vi "Begin.vi"(8 "error in":errorcluster) -> (0 "error out":errorcluster)   [LabVIEW 2017]
doc: "Called before other user functions, this VI is expected to open initial I/O refnums, load in file data, and do all program initialization. Notice that the <B>error out</B> terminal is simply used for data flow. Wiring it to other structures or subVIs ensures that this VI runs first."
uses:
  <vilib>/Rock Robotics/WPI/DriverStation/WPI_DriverStationRobotMode2.ctl
  <vilib>/Rock Robotics/WPI/Joystick/WPI_JoystickDeviceEnum.ctl
  <vilib>/Rock Robotics/WPI/Solenoid/WPI_SolenoidChannel.ctl
  <vilib>/Rock Robotics/SystemInterfaces/spilib/spi_bus.ctl
  C:/Users/Public/Documents/Cross The Road Electronics/Phoenix-LabVIEW/Motor Controller/Controls/CTRE_Phoenix_MotorControl_ControlMode.ctl
  <vilib>/Rock Robotics/WPI/ThirdParty/Phoenix-LabVIEW/Motor Controller/Controls/CTRE_Phoenix_MotorControl_NeutralMode.ctl
  <vilib>/Rock Robotics/WPI/ThirdParty/Phoenix-LabVIEW/Motor Controller/Controls/CTRE_Phoenix_MotorControl_FeedbackDevice.ctl
  <vilib>/Rock Robotics/SystemInterfaces/DIO/FPGA_DIOChannel.ctl
  <vilib>/Rock Robotics/SystemInterfaces/AI/FPGA_AIChannel.ctl
  Robot Global Data.vi
  <vilib>/Rock Robotics/WPI/Solenoid/WPI_SolenoidOpenDouble.vi
  <vilib>/Rock Robotics/WPI/Solenoid/WPI_SolenoidOpenSingle.vi
  <vilib>/Rock Robotics/WPI/Switch/WPI_SwitchOpenLimit.vi
  <vilib>/Rock Robotics/WPI/Gyro/WPI_GyroXRS450_SPI_Open.vi
  <vilib>/Rock Robotics/Network Tables/NT Write Numeric Array.vi
  <vilib>/Rock Robotics/Network Tables/NT Write String Array.vi
panel:
  in  "Right_P":dbl
  in  "Right_I":dbl
  in  "Right_D":dbl
  in  "Right_F":dbl
  in  "Left_F":dbl
  in  "Left_D":dbl
  in  "Left_I":dbl
  in  "Left_P":dbl
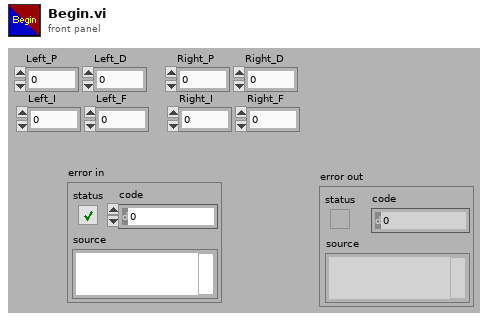
[diagram p1: front panel]
types:
  T1 = typedef "FPGA_AIChannel.ctl" = enum8{"AI 0", "AI 1", "AI 2", "AI 3", "AI MXP 0", "AI MXP 1", "AI MXP 2", "AI MXP 3", "Invalid"}
  T2 = typedef "FPGA_DIOChannel.ctl" = enum8{"DIO 0", "DIO 1", "DIO 2", "DIO 3", "DIO 4", "DIO 5", "DIO 6", "DIO 7", "DIO 8", "DIO 9", "DIO MXP 0", "DIO MXP 1", "DIO MXP 2", "DIO MXP 3", "DIO MXP 4", "DIO MXP 5", "DIO MXP 6", "DIO MXP 7", "DIO MXP 8", "DIO MXP 9", "DIO MXP 10", "DIO MXP 11", "DIO MXP 12", "DIO MXP 13", "DIO MXP 14", "DIO MXP 15", "SPI Port CS1", "SPI Port CS2", "SPI Port CS3", "SPI Port MISO", "SPI Port MOSI", "Invalid"}
  T3 = typedef "CTRE_Phoenix_MotorControl_FeedbackDevice.ctl" = i8
  T4 = typedef "CTRE_Phoenix_MotorControl_NeutralMode.ctl" = enum8{"EEPROMSetting", "Override to Coast", "Override to Brake"}
  T5 = typedef "CTRE_Phoenix_MotorControl_ControlMode.ctl" = u16
  T6 = typedef "spi_bus.ctl" = enum16{"SPI On-Board, CS0", "SPI On-Board, CS1", "SPI On-Board, CS2", "SPI On-Board, CS3", "SPI MXP", "Invalid"}
  T7 = typedef "WPI_SolenoidChannel.ctl" = enum8{"Solenoid 0", "Solenoid 1", "Solenoid 2", "Solenoid 3", "Solenoid 4", "Solenoid 5", "Solenoid 6", "Solenoid 7", "Invalid"}
  T8 = typedef "WPI_JoystickDeviceEnum.ctl" = enum16{"USB 0", "USB 1", "USB 2", "USB 3", "USB 4", "USB 5"}
  T9 = typedef "WPI_DriverStationRobotMode2.ctl" = enum16{"Autonomous Disabled", "Autonomous Enabled", "Teleop Disabled", "Teleop Enabled", "Disconnected", "Finish", "Test Disabled", "Test Enabled", "Emergency Stopped"}
  T10 = typedef "WPI_MotorControlDeviceRef.ctl" = cluster{"DeviceStatus":errorcluster, "Type":T11, "PWM":cluster{"PWM Channel":T12, "DeadBand":T13}, "CAN":cluster{"Device Number":u8, "SetOutput VI Ref":variant, "GetOutput VI Ref":variant, "Enable VI Ref":variant, "Disable VI Ref":variant, "Data":variant}, "Invert":bool, "DIO PWM":cluster{"PWM \"Enable\" Channel":T12, "DIOChannel":T2, "PWM Rate":dbl}}
  T11 = typedef "WPI_MotorControlType.ctl" = enum16{"PWM", "CAN", "DIO PWM"}
  T12 = typedef "FPGA_DIOPWMChannel.ctl" = enum8{"PWM 0", "PWM 1", "PWM 2", "PWM 3", "PWM 4", "PWM 5", "PWM 6", "PWM 7", "PWM 8", "PWM 9", "PWM MXP 0", "PWM MXP 1", "PWM MXP 2", "PWM MXP 3", "PWM MXP 4", "PWM MXP 5", "PWM MXP 6", "PWM MXP 7", "PWM MXP 8", "PWM MXP 9", "Invalid"}
  T13 = typedef "WPI_PWMDeadband.ctl" = cluster{"Name":string, "maxPositivePwm":i32, "minPositivePwm":i32, "centerPwm":i32, "maxNegativePwm":i32, "minNegativePwm":i32, "angularRange":u16}
  T14 = typedef "WPI_SolenoidDevRef.ctl" = cluster{"DevStatus":errorcluster, "Pneumatics Control Module":u8, "Forward Solenoid Channel":T7, "Reverse Solenoid Channel":T7}
  T15 = typedef "WPI_JoystickDevRef.ctl" = cluster{"Device":T8}
  T16 = typedef "WPI_AnalogChannelDevRef.ctl" = cluster{"DevStatus":errorcluster, "Analog Channel":T1}
  T17 = typedef "WPI_SwitchDevRef.ctl" = cluster{"DevStatus":errorcluster, "DIO Channel":T2, "CntIndex":T18, "Normally Closed":bool}
  T18 = typedef "FPGA_CounterCtrSystemIndex.ctl" = enum8{"Ctr 0", "Ctr 1", "Ctr 2", "Ctr 3", "Ctr 4", "Ctr 5", "Ctr 6", "Ctr 7", "Invalid"}
  T19 = typedef "WPI_GyroDevRef.ctl" = cluster{"DevStatus":errorcluster, "Analog Channel":T1, "Gain (VoltsPerDegree/Second)":dbl, "Gyro Type":enum16{"Analog", "XRS450"}, "Handle":i32, "SPI Bus":T6, "Device Found":bool, "Sample Rate":dbl, "Calibrate On Open":bool, "Offset":dbl}
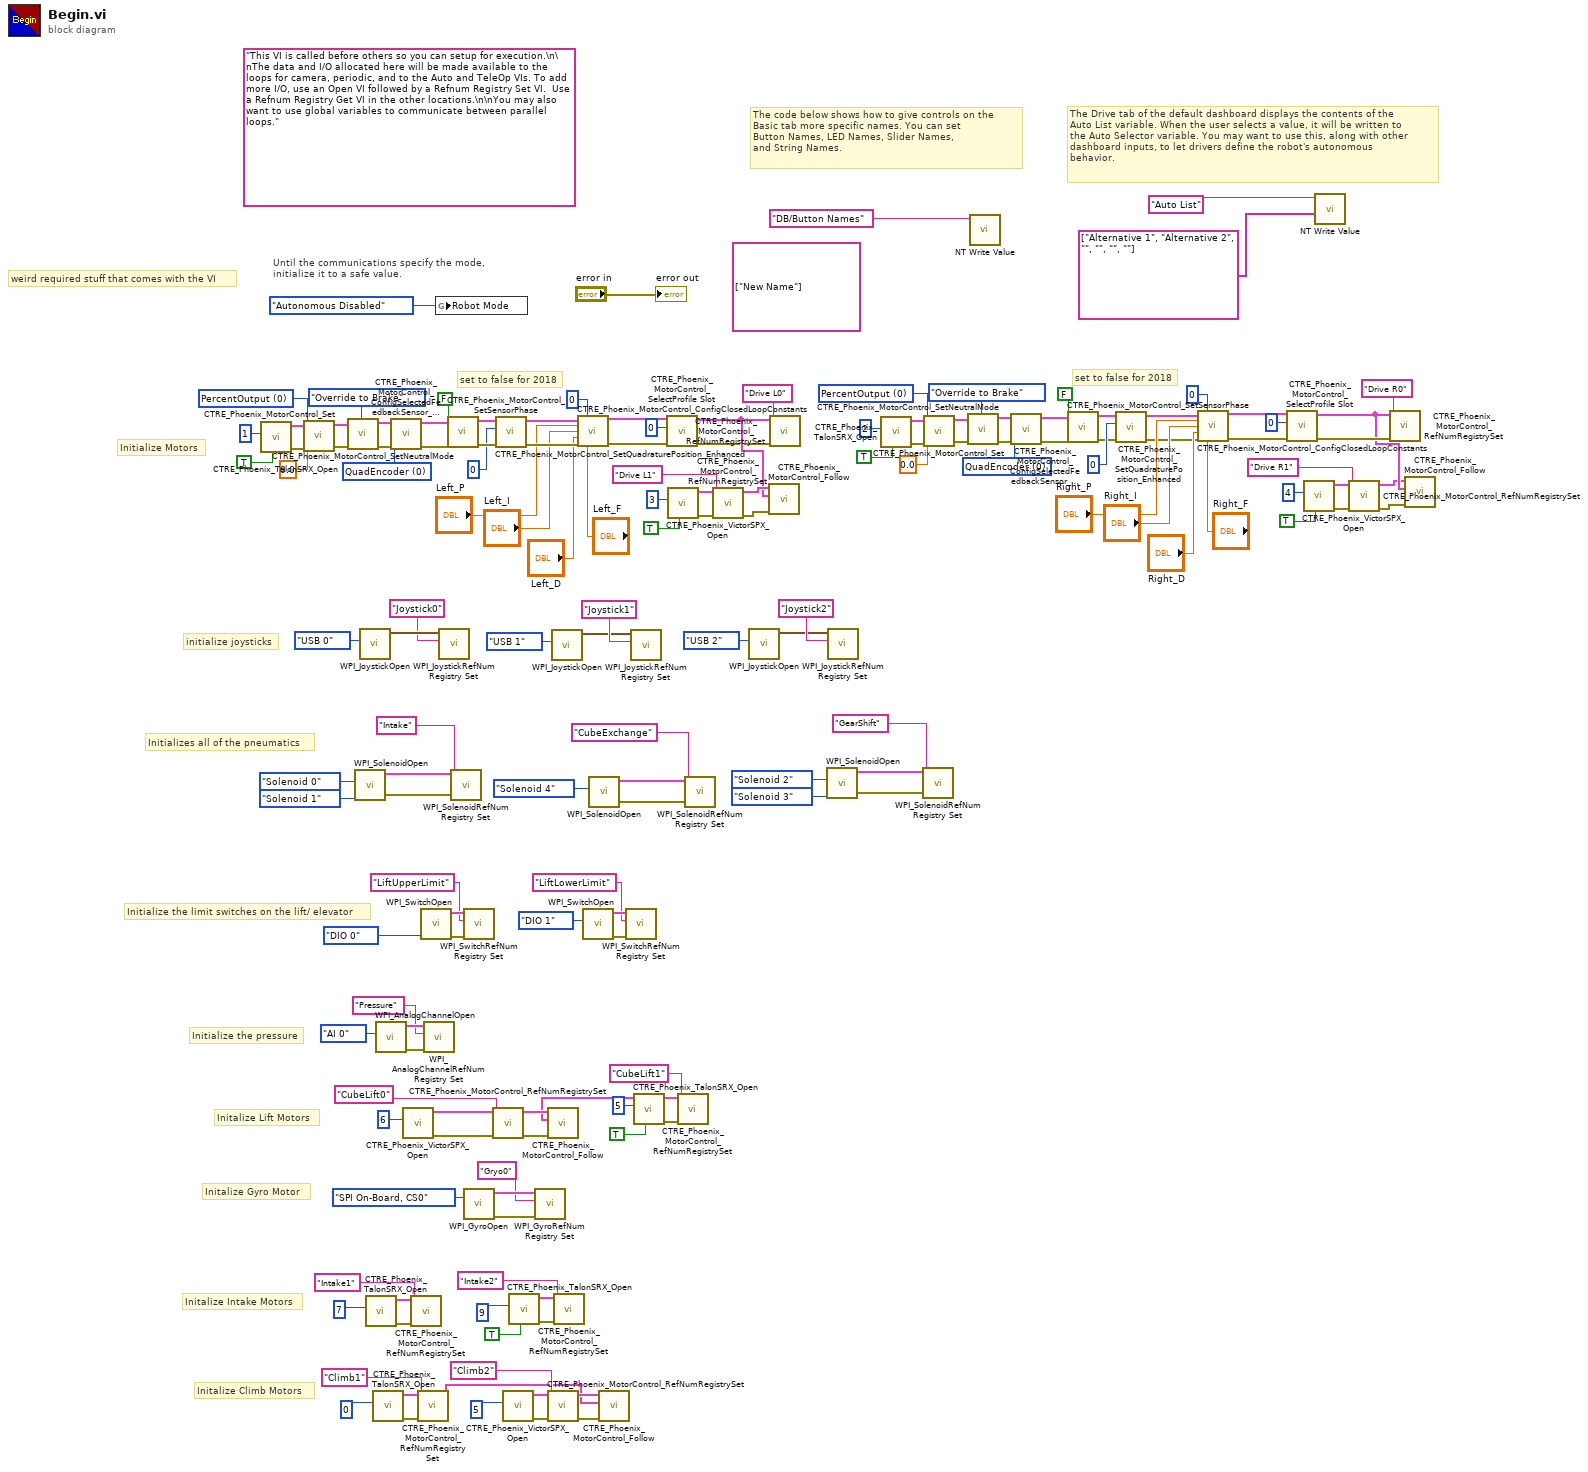
[diagram p0: block diagram]
diagram:
  w26 = T3 0 items=["None"=-1, "QuadEncoder"=0, "Analog"=2, "Tachometer"=4, "Pulse Width Encoded Position"=8, "Sensor Sum (S0 + S1)"=9, "Sensor Difference (D0 - D1)"=10, "Remote Source 0"=11, "Remote Source 1"=12, "Software Emulated"=15] ("Feedback Device")
  w21 = T5 0 items=["PercentOutput"=0, "Position"=1, "Velocity"=2, "Current"=3, "Follower"=5, "MotionProfile"=6, "MotionMagic"=7, "MotionMagicArc"=8, "MotionProfileArc"=10, "Disabled"=15] ("Control Mode")
  w63 = T3 0 items=["None"=-1, "QuadEncoder"=0, "Analog"=2, "Tachometer"=4, "Pulse Width Encoded Position"=8, "Sensor Sum (S0 + S1)"=9, "Sensor Difference (D0 - D1)"=10, "Remote Source 0"=11, "Remote Source 1"=12, "Software Emulated"=15] ("Feedback Device")
  w68 = T5 0 items=["PercentOutput"=0, "Position"=1, "Velocity"=2, "Current"=3, "Follower"=5, "MotionProfile"=6, "MotionMagic"=7, "MotionMagicArc"=8, "MotionProfileArc"=10, "Disabled"=15] ("Control Mode")
  (unwired) string[] ["New Name"]
  (unwired) "This VI is called before others so you can setup for execution.\n\nThe data and I/O allocated here will be made available to the loops for camera, periodic, and to the Auto and TeleOp VIs. To add more I/O, use an Open VI followed by a Refnum Registry Set VI.  Use a Refnum Registry Get VI in the other locations.\n\nYou may also want to use global variables to communicate between parallel loops."
  # "weird required stuff that comes with the VI"
  # "Initalize Climb Motors"
  # "Initalize Intake Motors"
  # "Initalize Gyro Motor"
  # "Initalize Lift Motors"
  # "Initialize the pressure"
  # "set to false for 2018"
  # "set to false for 2018"
  # "Initialize the limit switches on the lift/ elevator"
  # "Initializes all of the pneumatics"
  # "Initialize Motors"
  # "The Drive tab of the default dashboard displays the contents of the\nAuto List variable. When the user selects a value, it will be written to\nthe Auto Selector variable. You may want to use this, along with other\ndashboard inputs, to let drivers define the robot's autonomous\nbehavior."
  # "The code below shows how to give controls on the\nBasic tab more specific names. You can set\nButton Names, LED Names, Slider Names,\nand String Names."
  # "initialize joysticks"
  # "Until the communications specify the mode,\ninitialize it to a safe value."
  n1 = call "CTRE_Phoenix_TalonSRX_Open.vi"("Invert"=TRUE, "Device Number"=u8 1) -> ("error out"=w71:errorcluster, "CAN Talon SRX Ref"=w72:T10)  [unwired: 8 in]
  n2 = call <vilib>:"CTRE_Phoenix_MotorControl_Set.vi"("error in (no error)"=w71, "Output"=0.0, "Control Mode"=w68, "PhoenixMotorControlDevRef"=w72) -> ("error out"=w69:errorcluster, "PhoenixMotorControlDevRef"=w70:T10)  [unwired: 6 in]
  n3 = call <vilib>:"CTRE_Phoenix_MotorControl_SetNeutralMode.vi"("error in (no error)"=w69, "Motor Control Neutral Mode"=CTRE_Phoenix_MotorControl_NeutralMode."Override to Brake", "PhoenixMotorControlDevRef"=w70) -> ("error out"=w65:errorcluster, "PhoenixMotorControlDevRef"=w64:T10)  [unwired: 7 in]
  n4 = call-poly <vilib>:"WPI_SolenoidOpen.vi"("Reverse Solenoid Channel"=WPI_SolenoidChannel."Solenoid 1", "Forward Solenoid Channel"=WPI_SolenoidChannel."Solenoid 0") -> ("error out"=w114:errorcluster, "SolenoidDevRef"=w113:T14)  [unwired: 8 in]
  n5 = call <vilib>:"WPI_JoystickOpen.vi"("JoystickDevice"=WPI_JoystickDeviceEnum."USB 0") -> ("JoystickDevRef"=w142:T15)  [unwired: 10 in]
  n6 = call "CTRE_Phoenix_TalonSRX_Open.vi"("Device Number"=u8 7) -> ("error out"=w122:errorcluster, "CAN Talon SRX Ref"=w121:T10)  [unwired: 9 in]
  n7 = call "CTRE_Phoenix_TalonSRX_Open.vi"("Device Number"=u8 0) -> ("error out"=w135:errorcluster, "CAN Talon SRX Ref"=w134:T10)  [unwired: 9 in]
  n8 = call <vilib>:"WPI_AnalogChannelOpen.vi"("Analog Channel"=FPGA_AIChannel."AI 0") -> ("error out"=w4:errorcluster, "AIDeviceRef"=w3:T16)  [unwired: 9 in]
  n9 = call <vilib>:"CTRE_Phoenix_MotorControl_ConfigSelectedFeedbackSensor_Enhanced.vi"("error in (no error)"=w65, "Feedback Device"=w63, "PhoenixMotorControlDevRef"=w64) -> ("error out"=w61:errorcluster, "PhoenixMotorControlDevRef"=w62:T10)  [unwired: 7 in]
  n10 = call <vilib>:"CTRE_Phoenix_VictorSPX_Open.vi"("Device Number"=u8 6) -> ("error out"=w99:errorcluster, "CAN Talon SRX Ref"=w98:T10)  [unwired: 9 in]
  n11 = call "CTRE_Phoenix_MotorControl_RefNumRegistrySet.vi"("error in (no error)"=w122, "refnum name"="Intake1", "PhoenixMotorControlDevRef"=w121) -> ()  [unwired: 7 in, 2 out]
  n12 = call "CTRE_Phoenix_MotorControl_RefNumRegistrySet.vi"("error in (no error)"=w135, "refnum name"="Climb1", "PhoenixMotorControlDevRef"=w134) -> ("PhoenixMotorControlDevRef"=w82:T10)  [unwired: 7 in, 1 out]
  n13 = call-poly <vilib>:"WPI_SwitchOpen.vi"("DIO Channel"=FPGA_DIOChannel."DIO 0") -> ("error out"=w78:errorcluster, "SwitchDevRef"=w77:T17)  [unwired: 9 in]
  n14 = call <vilib>:"WPI_AnalogChannelRefNum Registry Set.vi"("error in (no error)"=w4, "refnum name"="Pressure", "AIDeviceRef"=w3) -> ()  [unwired: 7 in, 2 out]
  n15 = global write "Robot Global Data.vi" "Robot Mode"(WPI_DriverStationRobotMode2."Autonomous Disabled" ("Robot Mode")) -> ()
  n16 = call <vilib>:"WPI_JoystickRefNum Registry Set.vi"("refnum name"="Joystick0", "JoystickDevRef"=w142) -> ()  [unwired: 8 in, 2 out]
  n17 = call <vilib>:"CTRE_Phoenix_MotorControl_SetSensorPhase.vi"("error in (no error)"=w61, "PhaseSensor"=FALSE, "PhoenixMotorControlDevRef"=w62) -> ("error out"=w59:errorcluster, "PhoenixMotorControlDevRef"=w58:T10)  [unwired: 7 in]
  n18 = call <vilib>:"WPI_SolenoidRefNum Registry Set.vi"("error in (no error)"=w114, "refnum name"="Intake", "SolenoidDevRef"=w113) -> ()  [unwired: 7 in, 2 out]
  n19 = call <vilib>:"WPI_SwitchRefNum Registry Set.vi"("error in (no error)"=w78, "refnum name"="LiftUpperLimit", "SwitchDevRef"=w77) -> ()  [unwired: 7 in, 2 out]
  n20 = call-poly <vilib>:"WPI_GyroOpen.vi"("SPI Bus"=spi_bus."SPI On-Board, CS0") -> ("error out"=w91:errorcluster, "GyroDevRef"=w92:T19)  [unwired: 8 in, 1 out]
  n21 = call "CTRE_Phoenix_MotorControl_RefNumRegistrySet.vi"("error in (no error)"=w99, "refnum name"="CubeLift0", "PhoenixMotorControlDevRef"=w98) -> ("error out"=w87:errorcluster, "PhoenixMotorControlDevRef"=w86:T10)  [unwired: 7 in]
  n22 = call <vilib>:"CTRE_Phoenix_MotorControl_SetQuadraturePosition_Enhanced.vi"("error in (no error)"=w59, "New Position"=0, "PhoenixMotorControlDevRef"=w58) -> ("error out"=w53:errorcluster, "PhoenixMotorControlDevRef"=w56:T10)  [unwired: 7 in]
  n23 = call <vilib>:"CTRE_Phoenix_VictorSPX_Open.vi"("Device Number"=u8 5) -> ("error out"=w126:errorcluster, "CAN Talon SRX Ref"=w125:T10)  [unwired: 9 in]
  n24 = call "CTRE_Phoenix_TalonSRX_Open.vi"("Invert"=TRUE, "Device Number"=u8 9) -> ("error out"=w118:errorcluster, "CAN Talon SRX Ref"=w117:T10)  [unwired: 8 in]
  n25 = call <vilib>:"WPI_GyroRefNum Registry Set.vi"("error in (no error)"=w91, "refnum name"="Gryo0", "GyroDevRef"=w92) -> ()  [unwired: 7 in, 2 out]
  n26 = call "CTRE_Phoenix_MotorControl_RefNumRegistrySet.vi"("error in (no error)"=w126, "refnum name"="Climb2", "PhoenixMotorControlDevRef"=w125) -> ("error out"=w84:errorcluster, "PhoenixMotorControlDevRef"=w85:T10)  [unwired: 7 in]
  n27 = call <vilib>:"WPI_JoystickOpen.vi"("JoystickDevice"=WPI_JoystickDeviceEnum."USB 1") -> ("JoystickDevRef"=w150:T15)  [unwired: 10 in]
  n28 = call "CTRE_Phoenix_MotorControl_RefNumRegistrySet.vi"("error in (no error)"=w118, "refnum name"="Intake2", "PhoenixMotorControlDevRef"=w117) -> ()  [unwired: 7 in, 2 out]
  n29 = call <vilib>:"CTRE_Phoenix_MotorControl_ConfigClosedLoopConstants.vi"("PhoenixMotorControlDevRef"=w56, "slotIdx"=0, "P"="Left_P", "I"="Left_I", "D"="Left_D", "error in (no error)"=w53, "F"="Left_F") -> ("PhoenixMotorControlDevRef"=w55:T10, "error out"=w52:errorcluster)  [unwired: 7 in]
  n30 = call-poly <vilib>:"WPI_SwitchOpen.vi"("DIO Channel"=FPGA_DIOChannel."DIO 1") -> ("error out"=w75:errorcluster, "SwitchDevRef"=w74:T17)  [unwired: 9 in]
  n31 = call-poly <vilib>:"WPI_SolenoidOpen.vi"("Solenoid Channel"=WPI_SolenoidChannel."Solenoid 4" ("Forward Solenoid Channel")) -> ("error out"=w104:errorcluster, "SolenoidDevRef"=w103:T14)  [unwired: 9 in]
  n32 = call <vilib>:"CTRE_Phoenix_MotorControl_Follow.vi"("error in (no error)"=w84, "Master Controller to Follow"=w82, "PhoenixMotorControlDevRef"=w85) -> ()  [unwired: 7 in, 2 out]
  n33 = call <vilib>:"WPI_SwitchRefNum Registry Set.vi"("error in (no error)"=w75, "refnum name"="LiftLowerLimit", "SwitchDevRef"=w74) -> ()  [unwired: 7 in, 2 out]
  n34 = call <vilib>:"WPI_JoystickRefNum Registry Set.vi"("refnum name"="Joystick1", "JoystickDevRef"=w150) -> ()  [unwired: 8 in, 2 out]
  n35 = call "CTRE_Phoenix_TalonSRX_Open.vi"("Invert"=TRUE, "Device Number"=u8 5) -> ("error out"=w96:errorcluster, "CAN Talon SRX Ref"=w95:T10)  [unwired: 8 in]
  n36 = call <vilib>:"CTRE_Phoenix_MotorControl_SelectProfile Slot.vi"("error in (no error)"=w52, "slotIdx"=0, "PhoenixMotorControlDevRef"=w55) -> ("error out"=w51:errorcluster, "PhoenixMotorControlDevRef"=w54:T10)  [unwired: 7 in]
  n37 = call <vilib>:"CTRE_Phoenix_VictorSPX_Open.vi"("Invert"=TRUE, "Device Number"=u8 3) -> ("error out"=w131:errorcluster, "CAN Talon SRX Ref"=w130:T10)  [unwired: 8 in]
  n38 = call "CTRE_Phoenix_MotorControl_RefNumRegistrySet.vi"("error in (no error)"=w96, "refnum name"="CubeLift1", "PhoenixMotorControlDevRef"=w95) -> ("PhoenixMotorControlDevRef"=w83:T10)  [unwired: 7 in, 1 out]
  n39 = call <vilib>:"CTRE_Phoenix_MotorControl_Follow.vi"("error in (no error)"=w87, "Master Controller to Follow"=w83, "PhoenixMotorControlDevRef"=w86) -> ()  [unwired: 7 in, 2 out]
  n40 = call <vilib>:"WPI_SolenoidRefNum Registry Set.vi"("error in (no error)"=w104, "refnum name"="CubeExchange", "SolenoidDevRef"=w103) -> ()  [unwired: 7 in, 2 out]
  n41 = call "CTRE_Phoenix_MotorControl_RefNumRegistrySet.vi"("error in (no error)"=w131, "refnum name"="Drive L1", "PhoenixMotorControlDevRef"=w130) -> ("error out"=w128:errorcluster, "PhoenixMotorControlDevRef"=w127:T10)  [unwired: 7 in]
  n42 = call <vilib>:"WPI_JoystickOpen.vi"("JoystickDevice"=WPI_JoystickDeviceEnum."USB 2") -> ("JoystickDevRef"=w139:T15)  [unwired: 10 in]
  n43 = call <vilib>:"CTRE_Phoenix_MotorControl_Follow.vi"("error in (no error)"=w128, "Master Controller to Follow"=w54, "PhoenixMotorControlDevRef"=w127) -> ()  [unwired: 7 in, 2 out]
  n44 = call "CTRE_Phoenix_MotorControl_RefNumRegistrySet.vi"("error in (no error)"=w51, "refnum name"="Drive L0", "PhoenixMotorControlDevRef"=w54) -> ()  [unwired: 7 in, 2 out]
  n45 = call-poly <vilib>:"WPI_SolenoidOpen.vi"("Reverse Solenoid Channel"=WPI_SolenoidChannel."Solenoid 3", "Forward Solenoid Channel"=WPI_SolenoidChannel."Solenoid 2") -> ("error out"=w105:errorcluster, "SolenoidDevRef"=w106:T14)  [unwired: 8 in]
  n46 = call <vilib>:"WPI_JoystickRefNum Registry Set.vi"("refnum name"="Joystick2", "JoystickDevRef"=w139) -> ()  [unwired: 8 in, 2 out]
  n47 = call "CTRE_Phoenix_TalonSRX_Open.vi"("Invert"=TRUE, "Device Number"=u8 2) -> ("error out"=w18:errorcluster, "CAN Talon SRX Ref"=w17:T10)  [unwired: 8 in]
  n48 = call <vilib>:"WPI_SolenoidRefNum Registry Set.vi"("error in (no error)"=w105, "refnum name"="GearShift", "SolenoidDevRef"=w106) -> ()  [unwired: 7 in, 2 out]
  n49 = call <vilib>:"CTRE_Phoenix_MotorControl_Set.vi"("error in (no error)"=w18, "Output"=0.0, "Control Mode"=w21, "PhoenixMotorControlDevRef"=w17) -> ("error out"=w20:errorcluster, "PhoenixMotorControlDevRef"=w19:T10)  [unwired: 6 in]
  n50 = call <vilib>:"CTRE_Phoenix_MotorControl_SetNeutralMode.vi"("error in (no error)"=w20, "Motor Control Neutral Mode"=CTRE_Phoenix_MotorControl_NeutralMode."Override to Brake", "PhoenixMotorControlDevRef"=w19) -> ("error out"=w24:errorcluster, "PhoenixMotorControlDevRef"=w25:T10)  [unwired: 7 in]
  n51 = call-poly <vilib>:"NT Write Value.vi"("Name"="DB/Button Names") -> ()  [unwired: 10 in, 1 out]
  n52 = call <vilib>:"CTRE_Phoenix_MotorControl_ConfigSelectedFeedbackSensor_Enhanced.vi"("error in (no error)"=w24, "Feedback Device"=w26, "PhoenixMotorControlDevRef"=w25) -> ("error out"=w28:errorcluster, "PhoenixMotorControlDevRef"=w27:T10)  [unwired: 7 in]
  n53 = call <vilib>:"CTRE_Phoenix_MotorControl_SetSensorPhase.vi"("error in (no error)"=w28, "PhaseSensor"=FALSE, "PhoenixMotorControlDevRef"=w27) -> ("error out"=w30:errorcluster, "PhoenixMotorControlDevRef"=w31:T10)  [unwired: 7 in]
  n54 = call <vilib>:"CTRE_Phoenix_MotorControl_SetQuadraturePosition_Enhanced.vi"("error in (no error)"=w30, "New Position"=0, "PhoenixMotorControlDevRef"=w31) -> ("error out"=w36:errorcluster, "PhoenixMotorControlDevRef"=w33:T10)  [unwired: 7 in]
  n55 = call <vilib>:"CTRE_Phoenix_MotorControl_ConfigClosedLoopConstants.vi"("PhoenixMotorControlDevRef"=w33, "slotIdx"=0, "P"="Right_P", "I"="Right_I", "D"="Right_D", "error in (no error)"=w36, "F"="Right_F") -> ("PhoenixMotorControlDevRef"=w34:T10, "error out"=w37:errorcluster)  [unwired: 7 in]
  n56 = call <vilib>:"CTRE_Phoenix_MotorControl_SelectProfile Slot.vi"("error in (no error)"=w37, "slotIdx"=0, "PhoenixMotorControlDevRef"=w34) -> ("error out"=w38:errorcluster, "PhoenixMotorControlDevRef"=w35:T10)  [unwired: 7 in]
  n57 = call <vilib>:"CTRE_Phoenix_VictorSPX_Open.vi"("Invert"=TRUE, "Device Number"=u8 4) -> ("error out"=w10:errorcluster, "CAN Talon SRX Ref"=w11:T10)  [unwired: 8 in]
  n58 = call-poly <vilib>:"NT Write Value.vi"("String Array"=string[] ["Alternative 1", "Alternative 2", "", "", "", ""], "Name"="Auto List") -> ()  [unwired: 9 in, 1 out]
  n59 = call "CTRE_Phoenix_MotorControl_RefNumRegistrySet.vi"("error in (no error)"=w10, "refnum name"="Drive R1", "PhoenixMotorControlDevRef"=w11) -> ("error out"=w13:errorcluster, "PhoenixMotorControlDevRef"=w14:T10)  [unwired: 7 in]
  n60 = call "CTRE_Phoenix_MotorControl_RefNumRegistrySet.vi"("error in (no error)"=w38, "refnum name"="Drive R0", "PhoenixMotorControlDevRef"=w35) -> ()  [unwired: 7 in, 2 out]
  n61 = call <vilib>:"CTRE_Phoenix_MotorControl_Follow.vi"("error in (no error)"=w13, "Master Controller to Follow"=w35, "PhoenixMotorControlDevRef"=w14) -> ()  [unwired: 7 in, 2 out]
  "error out" <- "error in"
